vi "Get Shape.vi"(8 "error in (no error)":errorcluster, 11 "KD Tree in":refnum<class "KD Tree.lvclass">) -> (0 "error out":errorcluster, 2 "Shape":u32[](array[numeric]), 3 "KD Tree out":refnum<class "KD Tree.lvclass">)   [LabVIEW 2020, in "KD Tree.lvlib" / "KD Tree.lvclass"]
uses:
  KD Tree.lvclass
  KD Tree.lvlib
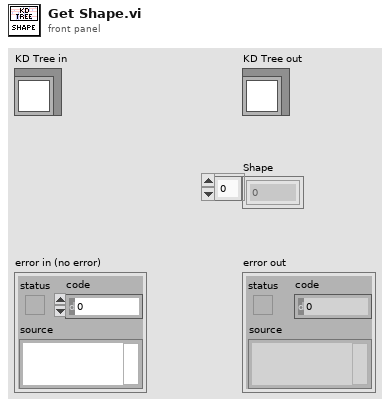
[diagram p1: front panel]
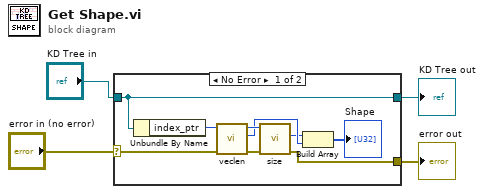
[diagram p0: block diagram]
diagram:
  n1 = case shown="No Error" "error in (no error)" {
    selector: "error in (no error)" -> [w11 w15]
    tunnel: [w9 w15] -> w3
    tunnel: [w13 w14] -> w1
    tunnel: "KD Tree in" -> [w13 w14]
    frame No Error {
      n2 = Unbundle By Name(w13) -> ("index_ptr"=w12:u64)
      n3 = call "veclen.vi"("error in (no error)"=w11, "index_ptr"=w12) -> ("error out"=w10:errorcluster, "Vector Length"=w7:u32, "index_ptr out"=w8:u64)  [unwired: 7 in]
      n4 = call "size.vi"("error in (no error)"=w10, "index_ptr"=w8) -> ("error out"=w9:errorcluster, "Index Dimensions"=w6:u32)  [unwired: 7 in, 1 out]
      n5 = Build Array(w6, w7) -> (→"Shape":u32[])
    }
    frame Error {
    }
  }
  "error out" <- w3
  "KD Tree out" <- w1
